vi "Watchdog Service.vi"(8 "error in (no error)":errorcluster, 11 "Watchdog Index":i32) -> (0 "error out":errorcluster, 3 "Watchdog Index Out":i32)   [LabVIEW 2013, in "RT Watchdog.lvlib"]
uses:
  RT Watchdog.lvlib
  Watchdog actions.ctl
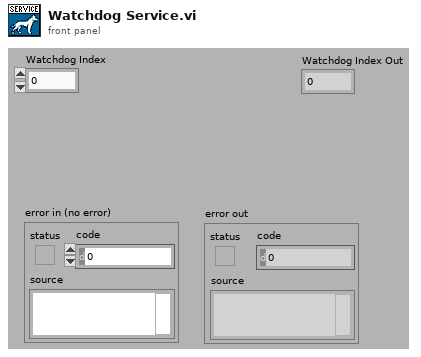
[diagram p1: front panel]
types:
  T1 = typedef "Watchdog actions.ctl" = enum16{"Init", "Enable", "Service", "Disable", "Check"}
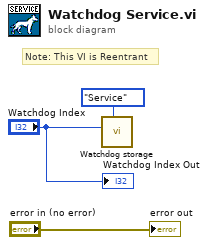
[diagram p0: block diagram]
diagram:
  # "Note: This VI is Reentrant"
  n1 = call "Watchdog storage.vi"("Command"=Watchdog_actions."Service", "Watchdog Index"="Watchdog Index") -> ()  [unwired: 7 in, 3 out]
  "error out" <- "error in (no error)"
  "Watchdog Index Out" <- "Watchdog Index"
